vi "PFI-28000-Chan-28144_Set Filter Cutoff HP.vi"(8 "error in (no error)":errorcluster, 10 "Filter Cutoff":dbl, 11 "PFI-28000-Chan-28144 in":refnum<class "PFI-28000-Chan-28144.lvclass">) -> (0 "error out":errorcluster, 3 "PFI-28000-Chan-28144 out":refnum<class "PFI-28000-Chan-28144.lvclass">)   [LabVIEW 2017, in "PFI-28000-Chan-28144.lvclass"]
uses:
  PFI-28000-Chan-28144.lvclass
  C:/wc/07143 Precision Filters 28000 Support/Driver/source/Channel/PFI-28000-Channel.lvclass
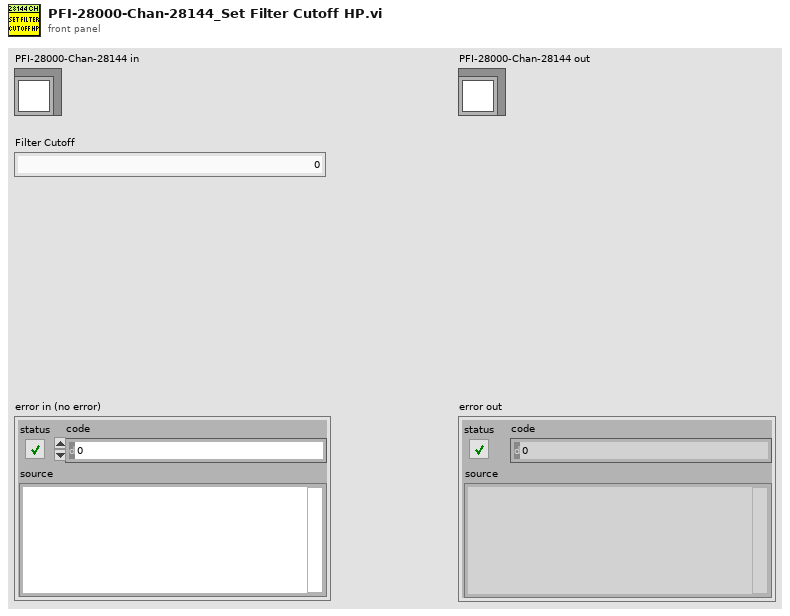
[diagram p1: front panel]
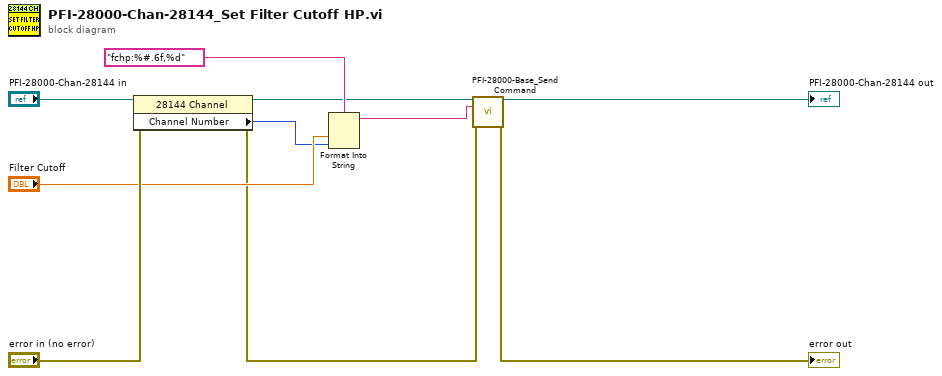
[diagram p0: block diagram]
diagram:
  n1 = property class="28144 Channel"(reference="PFI-28000-Chan-28144 in", error in="error in (no error)") -> (reference out=w5:refnum<class "PFI-28000-Chan-28144.lvclass">, error out=w2:errorcluster, "Channel Number"=w6:i32)
  n2 = Format Into String(format string="fchp:%#.6f,%d" ("empty string"), "Filter Cutoff", w6) -> (resulting string=w3:string)  [unwired: 2 in, 1 out]
  n3 = call-dynamic "PFI-28000-Base_Send Command.vi"("PFI-28000-Base in"=w5, "Command"=w3, "error in (no error)"=w2) -> ("PFI-28000-Base out"=→"PFI-28000-Chan-28144 out":refnum<class "PFI-28000-Chan-28144.lvclass">, "error out"=→"error out":errorcluster)  [unwired: 11 in]
